vi "Write SA Pin.vi"(8 "error in (no error)":errorcluster, 10 "SA Pin":string, 11 "SpecAn_AMPM in":refnum<class "SpecAn_AMPM.lvclass">) -> (0 "error out":errorcluster, 3 "SpecAn_AMPM out":refnum<class "SpecAn_AMPM.lvclass">)   [LabVIEW 2018, in "SeqAuto Evaluations.lvlib" / "SpecAn_AMPM.lvclass"]
uses:
  SpecAn_AMPM.lvclass
  SpecAn_AMPM.lvclass/SpecAn_AMPM.ctl
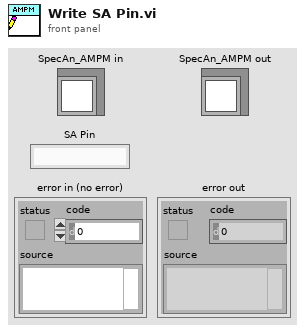
[diagram p1: front panel]
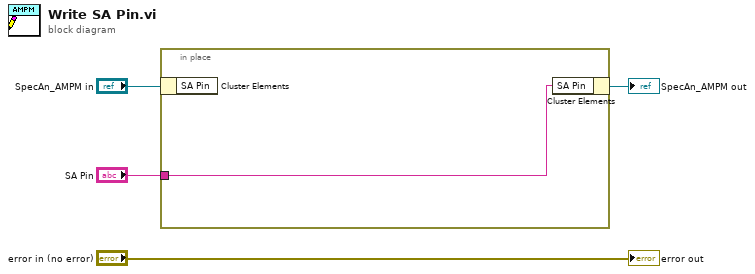
[diagram p0: block diagram]
diagram:
  n1 = in-place {
    in-place-border: "SA Pin" -> [w5]
    n2 = in-place-cluster #1("SpecAn_AMPM in") -> ()  [unwired: 1 out]
    n3 = in-place-cluster #1("SA Pin"=w5) -> (→"SpecAn_AMPM out":refnum<class "SpecAn_AMPM.lvclass">)
  }
  "error out" <- "error in (no error)"
